vi "Get Owning Path Default Value.vi"(0 "SG Path Group in":refnum<class "SG 18GHz Path Group.lvclass">, 11 "error in (no error)":errorcluster) -> (4 "SG Path Group out":refnum<class "SG 18GHz Path Group.lvclass">, 6 "Path":refnum<class "Path.lvclass">, 15 "error out":errorcluster)   [LabVIEW 2023, in "RFFixtureCharact.RFPM.lvlib" / "SG 18GHz Path Group.lvclass"]
uses:
  SG 18GHz Path Group.lvclass
  Common/Base Classes/Path/Path.lvclass
  Paths/SG Path/SG 18GHz Path.lvclass
  C:/srd-semi-rfcal-software/AuxTools/STSRFFixtureCharactUtility/Source/Code Modules/Common/Base Classes/Path/Path.lvclass
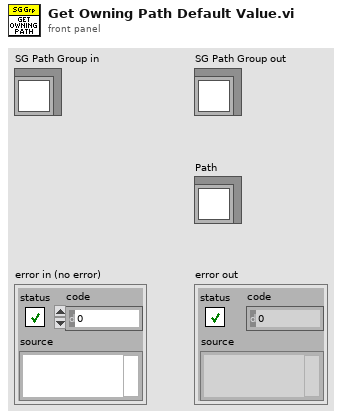
[diagram p1: front panel]
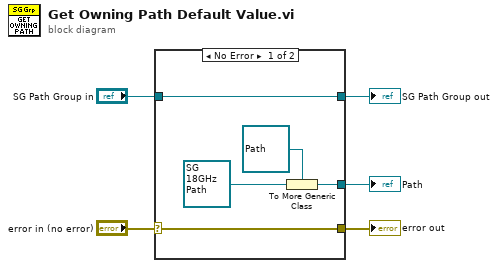
[diagram p0: block diagram]
diagram:
  n1 = case shown="No Error" "error in (no error)" {
    selector: "error in (no error)" -> [w7 w12]
    tunnel: [w8 _] -> w5
    tunnel: [w7 w12] -> w3
    tunnel: [w6 w11] -> w2
    tunnel: "SG Path Group in" -> [w6 w11]
    frame No Error {
      n2 = To More Generic Class(target class=refnum<class "Path.lvclass"> refnum ("Path"), reference=refnum<class "SG 18GHz Path.lvclass"> refnum ("STS Scalar Fixture Charact.lvlib:SG Path.lvclass")) -> (generic class reference=w8:refnum<class "Path.lvclass">)
    }
    frame Error {
    }
  }
  "error out" <- w3
  "SG Path Group out" <- w2
  "Path" <- w5
